vi "Delete DMA Channels.vi"(8 "error in (no error)":errorcluster, 10 "Input?":bool, 11 "Item Ref in":T1 format="%.0x") -> (0 "error out":errorcluster, 3 "Section Ref out":T1 format="%.0x")   [LabVIEW 2018, in "FPGA Addon System Explorer.lvlib"]
uses:
  FPGA Addon System Explorer.lvlib
  <vilib>/NI VeriStand/Custom Device Tools/Custom Device Utility Library/Custom Device Utility Library.lvlib
  <vilib>/NI VeriStand/Custom Device Tools/Custom Device Utility Library/NI VeriStand - Search for All Items by GUID.vi
  <vilib>/NI VeriStand/Custom Device API/Custom Device API.lvlib
  Addon Shared/SubVIs/Constants.vi
  Addon Shared/FPGA Addon Shared.lvlib
  <vilib>/NI VeriStand/Custom Device API/Custom Device Item Ref.ctl
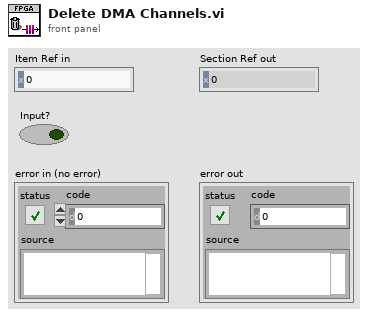
[diagram p1: front panel]
types:
  T1 = typedef "Custom Device API.lvlib/Custom Device Item Ref.ctl" = u64
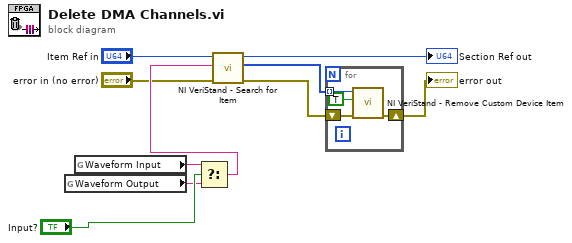
[diagram p0: block diagram]
diagram:
  n1 = global read "Constants.vi" "Waveform Output"() -> (w7:string)
  n2 = global read "Constants.vi" "Waveform Input"() -> (w8:string)
  n3 = Select(t=w8, s="Input?", f=w7) -> (s? t:f=w10:string)
  n4 = call-poly <vilib>:"NI VeriStand - Search for Item.vi"("error in"="error in (no error)", "Item GUID"=w10, "Section Ref in"="Item Ref in") -> ("error out"=w4:errorcluster, "Item Refs"=w1:T1[], "Section Ref out"=→"Section Ref out":T1)  [unwired: 5 in, 1 out]
  n5 = for {
    tunnel: w1 -> [w14] mode=indexing
    shift-right: [w12] -> w6
    shift-left: w4 -> [w13]
    n6 = call <vilib>:"NI VeriStand - Remove Custom Device Item.vi"("error in (no error)"=w13, "Force Delete (F)"=TRUE, "Item Ref in"=w14) -> ("error out"=w12:errorcluster)  [unwired: 7 in, 1 out]
  }
  "error out" <- w6
